vi "Config Data Close Reference.vi"(8 "error in (no error)":errorcluster caption="Fehler (Eingang, kein Fehler)", 11 "config data reference":T1 caption="Konfigurationsdaten-Referenz") -> (0 "error out":errorcluster caption="Fehler (Ausgang)")   [LabVIEW 2009]
doc: "Schließt eine Referenz auf ein Konfigurationsdaten-Objekt."
uses:
  <vilib>/Utility/config.llb/Config Data RefNum.ctl
  Config Data Registry Functions.ctl
  <vilib>/Utility/config.llb/NI_LVConfig.lvlib
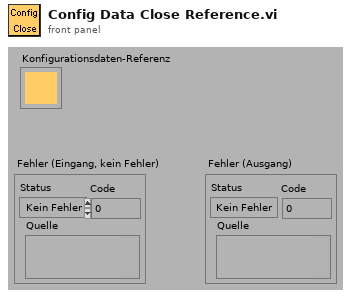
[diagram p1: front panel]
types:
  T1 = typedef "NI_LVConfig.lvlib/Config Data RefNum.ctl" = refnum<k1>
  T2 = typedef "Config Data Registry Functions.ctl" = enum16{"reset", "register", "get data", "get section", "set data", "unregister", "test", "get objects"}
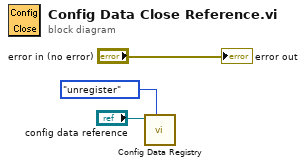
[diagram p0: block diagram]
diagram:
  n1 = call "Config Data Registry.vi"("function (get data)"=Config_Data_Registry_Functions."unregister", "config data"="config data reference") -> ()  [unwired: 3 in, 7 out]
  "error out" <- "error in (no error)"
